vi "CAN BL Excute.vi"(7 "Type":u32, 9 "NodeAddr":u16, 10 "CANIndex":i32, 11 "DevHandle":i32) -> (3 "function return":i32)   [LabVIEW 2010, in "usb2can.lvlib"]
doc: "int WINAPI CAN_BL_Excute(int DevHandle,int CANIndex,unsigned short NodeAddr,unsigned int Type);"
uses:
  usb2can.lvlib
  USB2XXX.dll
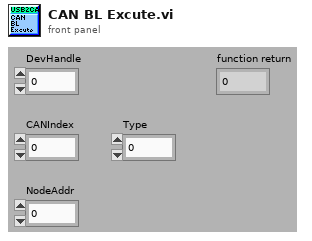
[diagram p1: front panel]
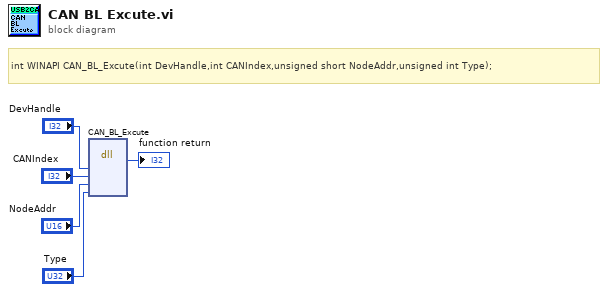
[diagram p0: block diagram]
diagram:
  # "int WINAPI CAN_BL_Excute(int DevHandle,int CANIndex,unsigned short NodeAddr,unsigned int Type);"
  n1 = dll-call lib="G:/OtherWork/USB2XXX_Example/trunk/Labview/PublicFiles/USB2XXX.*" fn="CAN_BL_Excute"("DevHandle"="DevHandle", "CANIndex"="CANIndex", "NodeAddr"="NodeAddr", "Type"="Type") -> (→"function return":i32)  [unwired: 7 in, 2 out]
